vi "QualityProblemHandling.vi"() -> ()   [LabVIEW 2015]
uses:
  GlobalPath.vi
  GlobalData.vi
panel:
  out "PanelName":string
  in  "Open Program 2":bool
  in  "New PCB ID":string
  in  "Old PCB ID":string
  in  "Done with saving ID?":bool
  in  "ptfe 4":bool caption="Scan the new PCB ID, enter it in the database and press SAVE"
  in  "ptfe 3":bool caption="Physically position the new PCB in place of the old one"
  in  "ptfe 2":bool caption="Go to the database under the current panel ID, select the faulty PCB\nand press \"Remove PCB\""
  # "When a PCB is below specs"
  # "Fill the following boxes:"
  # "At this point you need to re-take all the PCB measurements done so far\nThe following button will take you to the main panel where you need to select \"PCB Positioning\""
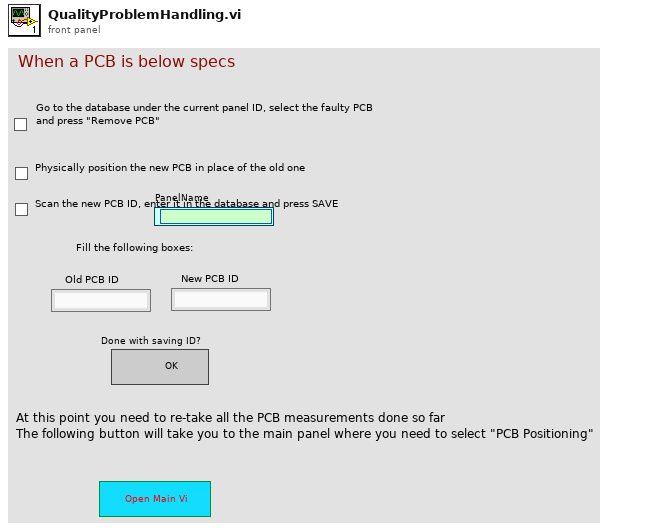
[diagram p1: front panel]
types:
  T1 = enum32{"Bad", "Idle", "Run top level", "Running"}
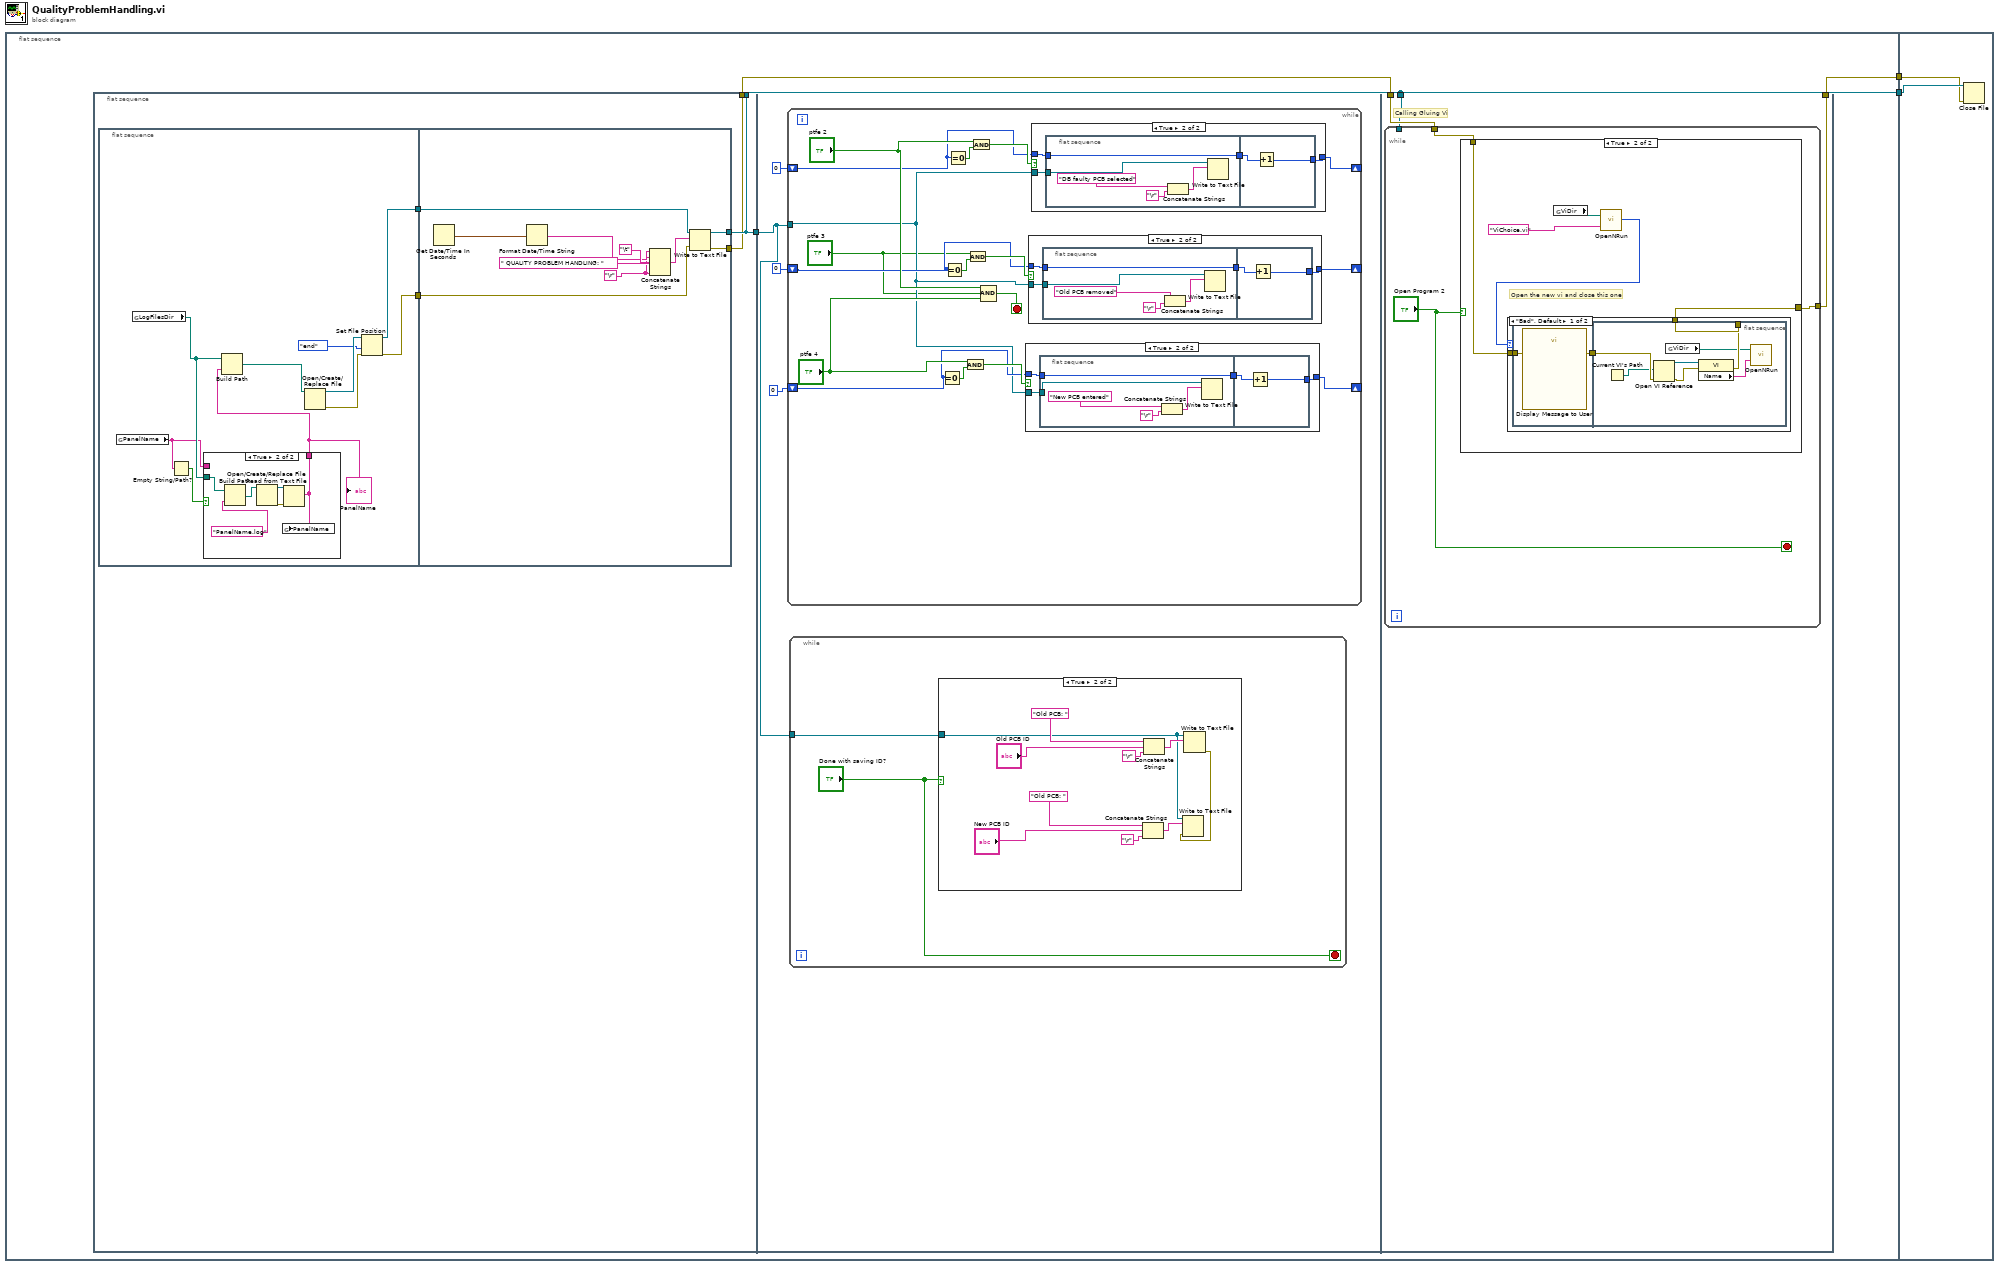
[diagram p0: block diagram]
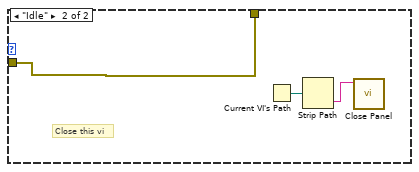
[diagram p8: hidden frame]
diagram:
  n1 = flat-sequence {
    tunnel: [w4] -> w2
    tunnel: [w3] -> w1
    tunnel: w2 -> [w135]
    tunnel: w1 -> [w134]
    frame #0 {
      n2 = flat-sequence {
        tunnel: [w9] -> w6
        tunnel: [w9] -> w4
        tunnel: [w8] -> w5
        tunnel: w6 -> [w38]
        tunnel: w5 -> [w109]
        tunnel: w4 -> [w108]
        tunnel: [w107] -> w3
        frame #0 {
          n3 = flat-sequence {
            tunnel: [w12] -> w10
            tunnel: [w11] -> w7
            tunnel: w10 -> [w33]
            tunnel: [w32] -> w9
            tunnel: [w31] -> w8
            tunnel: w7 -> [w30]
            frame #0 {
              n4 = global read "GlobalData.vi" "PanelName"() -> (w17:string)
              n5 = global read "GlobalPath.vi" "LogFilesDir"() -> (w20:path)
              n6 = Empty String/Path?(string/path=w17) -> (empty?=w18:bool)
              n7 = case shown="True" w18 {
                tunnel: w20 -> [_ w27]
                tunnel: [w21 w22] -> w19
                tunnel: w17 -> [w21 _]
                frame False {
                }
                frame True {
                  n8 = Build Path(base path=w27, name or relative path="PanelName.log") -> (appended path=w26:path)
                  n9 = Open/Create/Replace File(file path (use dialog)=w26) -> (refnum out=w23:refnum<file>, error out=w24:errorcluster)  [unwired: 5 in, 1 out]
                  n10 = Read from Text File(file (use dialog)=w23, error in=w24) -> (text=w22:string)  [unwired: 2 in, 3 out]
                  n11 = global write "GlobalData.vi" "PanelName"(w22) -> ()
                }
              }
              "PanelName" <- w19
              n12 = Build Path(base path=w20, name or relative path=w19) -> (appended path=w13:path)
              n13 = Open/Create/Replace File(file path (use dialog)=w13) -> (refnum out=w16:refnum<file>, error out=w15:errorcluster)  [unwired: 5 in, 1 out]
              n14 = Set File Position(refnum=w16, from (0:start)=enum16{"start", "end", "current"}."end", error in=w15) -> (refnum out=w12:refnum<file>, error out=w11:errorcluster)  [unwired: 1 in]
            }
            frame #1 {
              w28 = "\r"
              n15 = Get Date/Time In Seconds() -> (seconds since 1Jan1904=w29:timestamp)
              n16 = Format Date/Time String(seconds (now)=w29) -> (date/time string=w35:string)  [unwired: 2 in]
              n17 = Concatenate Strings(w28, w35, "\t", " QUALITY PROBLEM HANDLING: ", w28) -> (w34:string)
              n18 = Write to Text File(file (use dialog)=w33, text=w34, error in=w30) -> (refnum out=w32:refnum<file>, error out=w31:errorcluster)  [unwired: 1 in, 1 out]
            }
          }
        }
        frame #1 {
          n19 = while {
            tunnel: w38 -> [w55]
            shift-right: [w65] -> _
            shift-left: 0 -> [w66]
            shift-right: [w61] -> _
            shift-left: 0 -> [w62]
            shift-right: [w56] -> _
            shift-left: 0 -> [w57]
            stop <- w70 stop-if-true
            n20 = Equal To 0?(x=w57) -> (x = 0?=w60:bool)
            n21 = Equal To 0?(x=w62) -> (x = 0?=w64:bool)
            n22 = Equal To 0?(x=w66) -> (x = 0?=w69:bool)
            n23 = And(x="ptfe 4", y=w60) -> (x .and. y?=w59:bool)
            n24 = And(x="ptfe 3", y=w64) -> (x .and. y?=w63:bool)
            n25 = And(x="ptfe 2", y=w69) -> (x .and. y?=w68:bool)
            n26 = Compound Arithmetic op=AND("ptfe 2", "ptfe 3", "ptfe 4") -> (w70:bool)
            n27 = case shown="True" w59 {
              tunnel: w55 -> [_ w75]
              tunnel: w57 -> [w71 w73]
              tunnel: [w71 w72] -> w56
              frame False {
              }
              frame True {
                n28 = flat-sequence {
                  tunnel: w75 -> [w78]
                  tunnel: [w77] -> w74
                  tunnel: w73 -> [w77]
                  tunnel: w74 -> [w82]
                  tunnel: [w81] -> w72
                  frame #0 {
                    n29 = Concatenate Strings("New PCB entered", "\r") -> (w80:string)
                    n30 = Write to Text File(file (use dialog)=w78, text=w80) -> ()  [unwired: 2 in, 3 out]
                  }
                  frame #1 {
                    n31 = Increment(x=w82) -> (x+1=w81:i32)
                  }
                }
              }
            }
            n32 = case shown="True" w63 {
              tunnel: w55 -> [_ w87]
              tunnel: w62 -> [w83 w85]
              tunnel: [w83 w84] -> w61
              frame False {
              }
              frame True {
                n33 = flat-sequence {
                  tunnel: w87 -> [w90]
                  tunnel: [w89] -> w86
                  tunnel: w85 -> [w89]
                  tunnel: w86 -> [w94]
                  tunnel: [w93] -> w84
                  frame #0 {
                    n34 = Concatenate Strings("Old PCB removed", "\r") -> (w92:string)
                    n35 = Write to Text File(file (use dialog)=w90, text=w92) -> ()  [unwired: 2 in, 3 out]
                  }
                  frame #1 {
                    n36 = Increment(x=w94) -> (x+1=w93:i32)
                  }
                }
              }
            }
            n37 = case shown="True" w68 {
              tunnel: w55 -> [_ w99]
              tunnel: w66 -> [w95 w97]
              tunnel: [w95 w96] -> w65
              frame False {
              }
              frame True {
                n38 = flat-sequence {
                  tunnel: w99 -> [w102]
                  tunnel: [w101] -> w98
                  tunnel: w97 -> [w101]
                  tunnel: w98 -> [w106]
                  tunnel: [w105] -> w96
                  frame #0 {
                    n39 = Concatenate Strings("DB faulty PCB selected", "\r") -> (w104:string)
                    n40 = Write to Text File(file (use dialog)=w102, text=w104) -> ()  [unwired: 2 in, 3 out]
                  }
                  frame #1 {
                    n41 = Increment(x=w106) -> (x+1=w105:i32)
                  }
                }
              }
            }
          }
          n42 = while {
            tunnel: w38 -> [w42]
            stop <- "Done with saving ID?" stop-if-true
            n43 = case shown="True" "Done with saving ID?" {
              tunnel: w42 -> [_ w44]
              frame False {
              }
              frame True {
                n44 = Concatenate Strings("Old PCB: ", "New PCB ID", "\r") -> (w49:string)
                n45 = Concatenate Strings("Old PCB: ", "Old PCB ID", "\r") -> (w53:string)
                n46 = Write to Text File(file (use dialog)=w44, text=w53) -> (error out=w45:errorcluster)  [unwired: 2 in, 2 out]
                n47 = Write to Text File(file (use dialog)=w44, text=w49, error in=w45) -> ()  [unwired: 1 in, 3 out]
              }
            }
          }
        }
        frame #2 {
          # "Calling Gluing Vi"
          n48 = while {
            tunnel: w109 -> [w112]
            tunnel: [w111] -> w107
            tunnel: w108 -> [_]
            stop <- "Open Program 2" stop-if-true
            n49 = case shown="True" "Open Program 2" {
              tunnel: w112 -> [w113 w115]
              tunnel: [w113 w114] -> w111
              frame False {
              }
              frame True {
                # "Open the new vi and close this one"
                n50 = global read "GlobalPath.vi" "ViDir"() -> (w118:path)
                n51 = call "OpenNRun.vi"("VI name"="ViChoice.vi", "ViDirPath"=w118) -> ("Execution:State"=w117:T1)
                n52 = case shown="\"Bad\", Default" w117 {
                  tunnel: [w121 w133] -> w114
                  tunnel: w115 -> [w120 w133]
                  frame "Bad", Default {
                    n53 = flat-sequence {
                      tunnel: w120 -> [w122]
                      tunnel: [w123] -> w119
                      tunnel: [w127] -> w121
                      tunnel: w119 -> [w126]
                      frame #0 {
                        n54 = call "Display Message to User"("error in (no error)"=w122) -> ("error out"=w123:errorcluster)  [unwired: 9 in, 1 out]
                      }
                      frame #1 {
                        n55 = Current VI's Path() -> (path=w124:path)
                        n56 = Open VI Reference(vi path=w124, error in (no error)=w126) -> (vi reference=w130:refnum<vi>, error out=w129:errorcluster)  [unwired: 4 in]
                        n57 = global read "GlobalPath.vi" "ViDir"() -> (w125:path)
                        n58 = property class="VI"(reference=w130, error in=w129) -> (error out=w127:errorcluster, "Name"=w128:string)  [unwired: 1 out]
                        n59 = call "OpenNRun.vi"("VI name"=w128, "ViDirPath"=w125) -> ()  [unwired: 1 out]
                      }
                    }
                  }
                  frame "Idle" {
                    # "Close this vi"
                    n60 = Current VI's Path() -> (path=w132:path)
                    n61 = Strip Path(path=w132) -> (name=w131:string)  [unwired: 1 out]
                    n62 = call <vilib>:"Close Panel.vi"("VI name"=w131) -> ()  [unwired: 10 in, 1 out]
                  }
                }
              }
            }
          }
        }
      }
    }
    frame #1 {
      n63 = Close File(refnum=w135, error in=w134) -> ()  [unwired: 2 out]
    }
  }
